vi "AB_ProgressBar_Fire_New_Item.vi"(8 "error in (no error)":errorcluster, 10 "Label":string, 11 "progressBarEvents in":T1) -> (0 "error out":errorcluster, 3 "progressBarEvents out":T1)   [LabVIEW 2020]
uses:
  <resource>/Framework/Providers/Common/provcom_ProgressBar_Events.ctl
  <resource>/Framework/Providers/API/mxLvBuildError.ctl
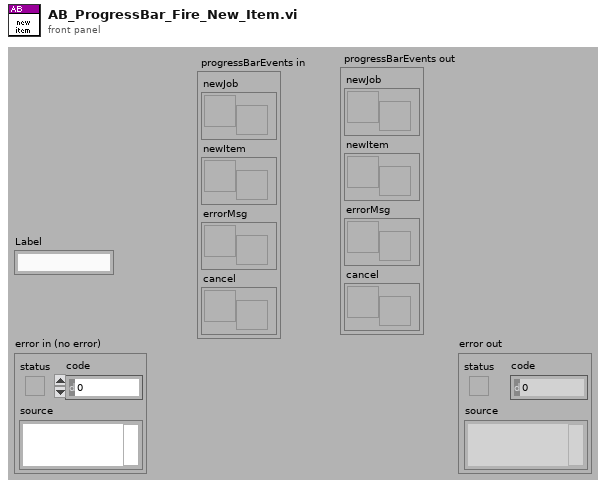
[diagram p1: front panel]
types:
  T1 = typedef "provcom_ProgressBar_Events.ctl" = cluster{"newJob":refnum<user-event>, "newItem":refnum<user-event>, "errorMsg":T2, "cancel":refnum<user-event>}
  T2 = typedef "mxLvBuildError.ctl" = refnum<user-event>
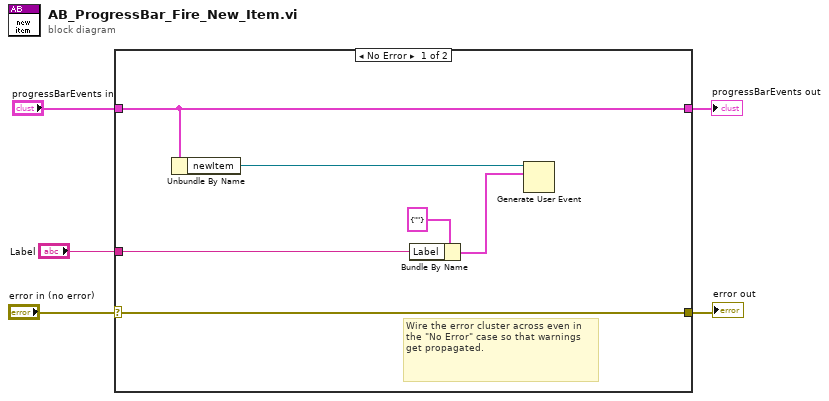
[diagram p0: block diagram]
diagram:
  n1 = case shown="No Error" "error in (no error)" {
    selector: "error in (no error)" -> [w11 w13]
    tunnel: [w11 w13] -> w4
    tunnel: [w10 w12] -> w2
    tunnel: "progressBarEvents in" -> [w10 w12]
    tunnel: "Label" -> [w6 _]
    frame No Error {
      # "Wire the error cluster across even in the \"No Error\" case so that warnings get propagated."
      n2 = Unbundle By Name(w10) -> ("newItem"=w7:refnum<user-event>)
      n3 = Bundle By Name(cluster=cluster{"Label":string} {"Label"=""} ("event data"), "Label"=w6) -> (w8:cluster{"Label":string})
      n4 = Generate User Event(user event=w7, event data cluster=w8) -> ()  [unwired: 2 in, 2 out]
    }
    frame Error {
    }
  }
  "error out" <- w4
  "progressBarEvents out" <- w2
